vi "DRR_Query.vi"(0 "System no.":i32=1 min=1 max=4 step=1, 2 "Rec. table IDs":i32[](array[numeric]), 3 "Without parameter?":bool, 5 "error in":errorcluster, 6 "Xo":i32=1, 7 "N":i32=100, 8 "Nmax":i32=1024, 12 "Stop refnum":refnum<vi>) -> (14 "Data":dbl[][](array[numeric]) format="%.2f", 15 "Names":string[](array[string]), 16 "Sample Time":dbl format="%.10f", 17 "DRR? string":string, 19 "error out":errorcluster)   [LabVIEW 2020]
doc: "Returns N recorded data points. If N is greater than Nmax, multiple queries are sent. For large Nmax values, communication timeout must be set long enough, otherwise a communication error may occur.\n\nAnalog: Rec. table IDs, x0, N and Nmax are not valid. Without parameter? must be TRUE.\n\nC-413: X0 >= 1. Nmax = 4096. The 4096 points are in equal shares assigned to the available data recorder tables. By default, the number of tables is 8. It can be reduced by setting the appropriate parameter value, see C-413 user manual for details.\n\nC-702: Nmax = 262144. X0 >= 0.\n\nC-843: X0 >= 1. Check C-843 user manual for valid Nmax values. Some hardware revisions don't allow the parallel use of DIO and the data recorder. To switch between both modes the C-843 needs to be reconnected. The number of tables is 4. The available points are in equal shares assigned to the available data recorder tables. By default, the number of tables is 4. It can be reduced with DRC, see C-843 user manual for details. If N = -1 all points of the last record are returned.\n\nC-866: X0 >= 1. Nmax = 32,256. If N = -1 all points of the last record are returned.\n\nC-867: X0 >= 1. Nmax = 8192. The number of tables is 4.\n\nC-877: Xo >= 1. Nmax = 8192.The number of tables is 4.\n\nC-884: Xo >= 1. Nmax = 8192. The number of tables is 8.\n\nC-891: Xo >= 1. Nmax = 16384.The C-891 has four data recorder tables with 4096 points per table. It can be changed to 1, 2 or 8 by setting the appropriate parameter value, see user manual for details.\n\nE-517, E-518: X0 >= 1. Nmax = 8192. The number of tables is 3.\n\nE-709: Xo >= 1. Nmax = 4096. The 4096 points are in equal shares assigned to the available data recorder tables. By default, the number of tables is 4. It can be reduced by setting the appropriate parameter value, see E-709 user manual for details.\n\nE-710: X0 >= 1. Nmax = 32,256.\n\nE-712: X0 >= 1. Nmax = 262,144. The 262,144 points are in equal shares assigned to the available data recorder tables. By default, the number of tables is 8. It can be reduced by setting the appropriate parameter value, see E-712 user manual for details.\n\nE-725, E-727: X0 >= 1. Nmax = 262,144. The 262,144 points are in equal shares assigned to the available data recorder tables. By default, the number of tables is 8. It can be reduced by setting the appropriate parameter value, see controller user manual for details. \n\nE-753: X0 >= 1. Nmax = 65,536. The 65,536 points are in equal shares assigned to the available data recorder tables. By default, the number of tables is 8. It can be reduced by setting the appropriate parameter value, see controller user manual for details.\nE-754: X0 >= 1. Nmax = 1,048,576. The 1,048,576 points are in equal shares assigned to the available data recorder tables. By default, the number of tables is 8. It can be reduced by setting the appropriate parameter value, see E-754 user manual for details.\n\nE-755: X0 >= 1. Nmax = 4,096.\n\nE-761: X0 >= 0. Recording takes place for all recorder tables as long as the wave generator is running for an arbitrary axis, when an impulse is started with IMP or when a step is started with STE. The assignment of axis and data sources to the recorder tables is as follows:\ntable 1: axis 1 actual position\ntable 2: axis 2 actual position\ntable 3: axis 3 actual position\ntable 4: analog input voltage (same value as read with TAV?, i.e. contains gain and offset for the analog input, see E-761 user manual).\nThe maximum number of data points is 8192 per recorder table.\n\nE-861: X0 >= 1. Nmax = 1024. Two data recorder tables with 1024 points per table are provided.\n\nE-871, E-873, E-874: Xo >= 1. Nmax = 1024. The number of tables is 2.\n\nC-887, F-206: Xo >= 1. See controller user manual for Nmax default value (can be changed with SPA.vi). Only for GCS syntax version = GCS 2.0 or higher (check with CSV?.vi. If CSV?.vi is not supported, syntax version is GCS 1.0). See controller user manual for available data recorder tables and points. \n\nC-887, M-8X0: For GCS syntax version = 1.0 (Check with CSV?.vi. If CSV?.vi is not supported, syntax version is GCS 1.0), Rec. table IDs, xo, N and Nmax are not valid and Without parameter? must be TRUE. \nFor GCS syntax version = 2.0, Xo >= 1. See controller user manual for available data recorder tables and points. The maximum number of points to be recorded per table (Nmax) can be changed with SPA.vi .\nOnly supported if controller is based on C-842.80 board or GCS syntax version = GCS 2.0 or higher (Check with CSV?.vi. If CSV?.vi is not supported, syntax version is GCS 1.0). For GCS 1.0, returns 360 motor current values recorded during execution of DRV. \n\nMercury_GCS: Xo >= 1. Nmax = 1024. See controller user manual for available data recorder tables."
panel:
  in  "Local stop":bool
  # "Returns N recorded data points. If N is greater than Nmax, multiple queries are sent. For large\nNmax values, communication timeout must be set long enough, otherwise a comm.error may\noccur."
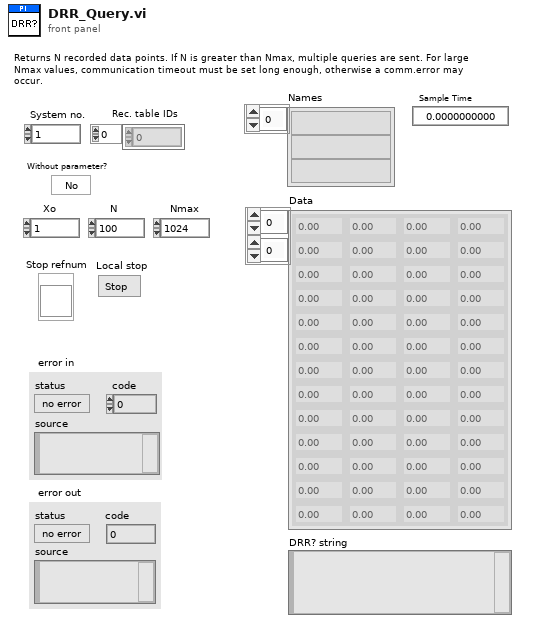
[diagram p1: front panel]
types:
  T1 = cluster{"Read (F)/Write":bool, "Path":path, "Datastream":string, "ArrayName":string}
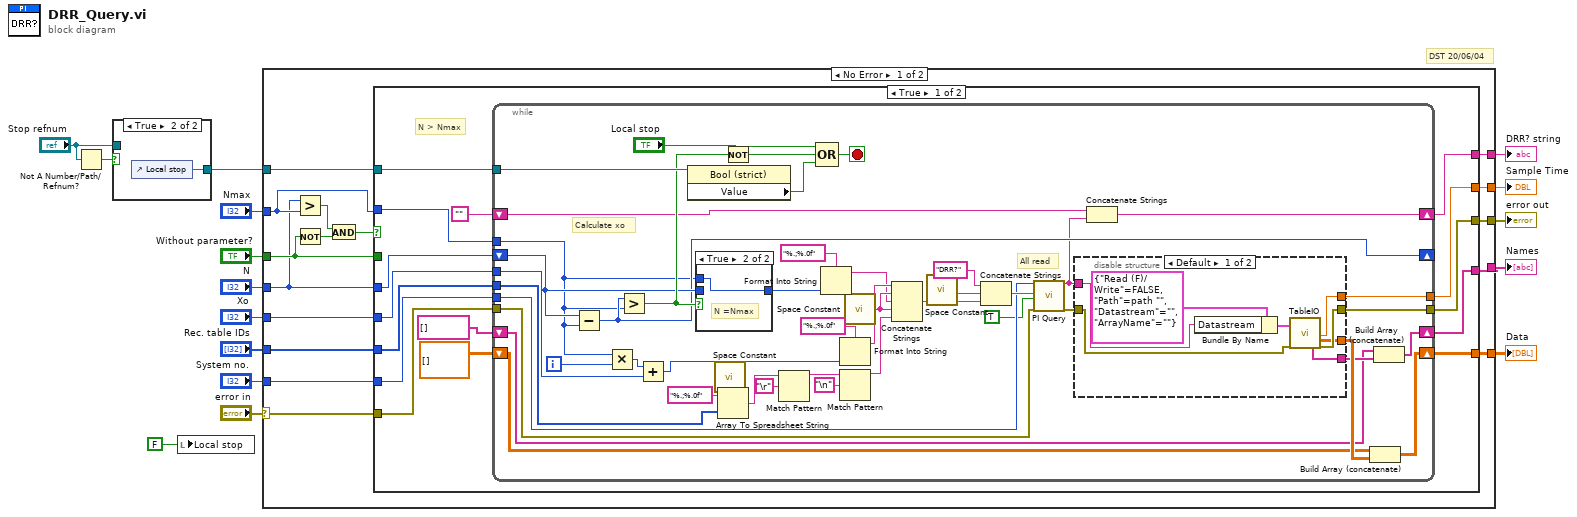
[diagram p0: block diagram]
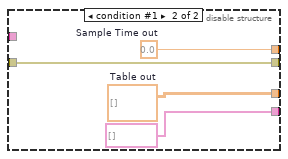
[diagram p3: hidden frame]
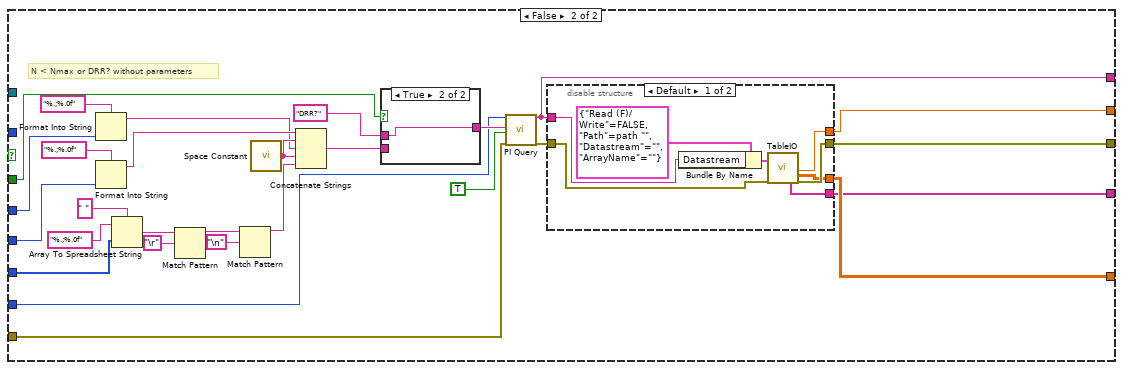
[diagram p5: hidden frame]
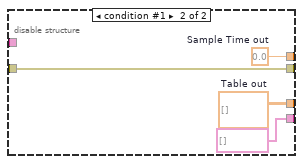
[diagram p6: hidden frame]
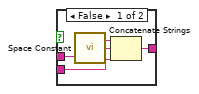
[diagram p7: hidden frame]
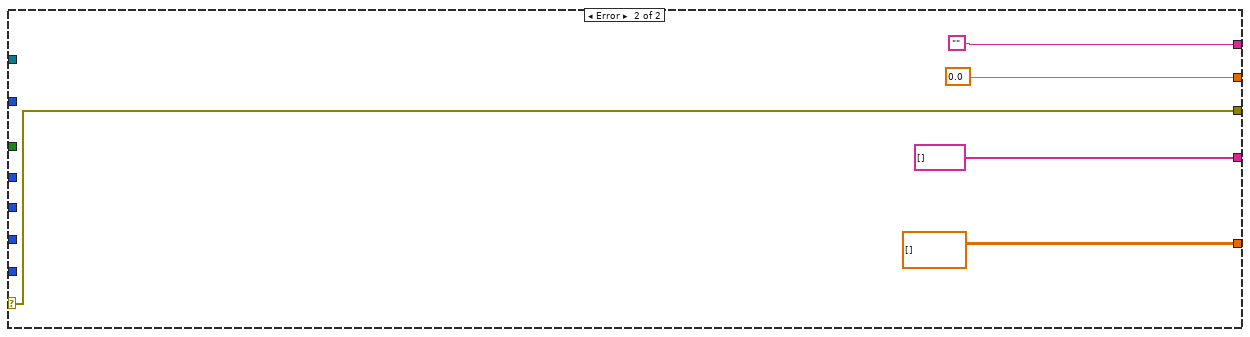
[diagram p8: hidden frame]
diagram:
  # "DST 20/06/04"
  n1 = Not A Number/Path/Refnum?(number/path/refnum="Stop refnum") -> (NaN/Path/Refnum?=w6:bool)
  n2 = case shown="True" w6 {
    tunnel: [w17 w18] -> w3
    tunnel: "Stop refnum" -> [w17 _]
    frame False {
    }
    frame True {
      n3 = control-ref of="Local stop"() -> (w18:refnum<vi>)
    }
  }
  n4 = local write "Local stop"(FALSE ("Local stop")) -> ()
  n5 = case shown="No Error" "error in" {
    selector: "error in" -> [w19 w155]
    tunnel: "System no." -> [w34 _]
    tunnel: "Rec. table IDs" -> [w28 _]
    tunnel: [w33 w155] -> w15
    tunnel: [w32 dbl[][] [] ("Table out")] -> w11
    tunnel: "N" -> [w24 _]
    tunnel: "Xo" -> [w31 _]
    tunnel: "Nmax" -> [w26 _]
    tunnel: [w30 0.0 ("Sample Time out")] -> w10
    tunnel: [w29 string[] [] ("Names out")] -> w9
    tunnel: "Without parameter?" -> [w25 _]
    tunnel: w3 -> [w27 _]
    tunnel: [w20 ""] -> w2
    frame No Error {
      n6 = Greater?(x=w24, y=w26) -> (0:w23:bool)
      n7 = Not(x=w25) -> (.not. x?=w22:bool)
      n8 = And(x=w23, y=w22) -> (x .and. y?=w21:bool)
      n9 = case shown="True" w21 {
        tunnel: w34 -> [w49 w135]
        tunnel: [w48 w133] -> w33
        tunnel: [w47 w132] -> w32
        tunnel: w31 -> [w46 w130]
        tunnel: w19 -> [w45 w128]
        tunnel: w24 -> [w44 w127]
        tunnel: [w43 w126] -> w30
        tunnel: [w42 w125] -> w29
        tunnel: w28 -> [w41 w119]
        tunnel: w25 -> [_ w116]
        tunnel: w27 -> [w40 _]
        tunnel: w26 -> [w39 _]
        tunnel: [w36 w111] -> w20
        frame True {
          # "N > Nmax"
          n10 = while {
            tunnel: w49 -> [w93]
            tunnel: [w91] -> w48
            tunnel: w46 -> [w54]
            tunnel: w45 -> [w88]
            tunnel: w41 -> [w81]
            tunnel: w40 -> [w74]
            shift-right: [w68] -> _
            shift-left: w44 -> [w69]
            shift-right: [w65] -> w47
            shift-left: dbl[][] [] -> [w66]
            shift-right: [w63] -> w42
            shift-left: string[] [] -> [w62]
            tunnel: w39 -> [w50]
            tunnel: [w87] -> w43
            shift-right: [w59] -> w36
            shift-left: "" -> [w60]
            i -> [w51]
            stop <- w72 stop-if-true
            # "All read"
            # "Calculate xo"
            n11 = Subtract(x=w69, y=w50) -> (x-y=w68:i32)
            n12 = Multiply(x=w50, y=w51) -> (x*y=w52:i32)
            n13 = Greater?(x=w68, y=w50) -> (0:w70:bool)
            n14 = Add(x=w52, y=w54) -> (x+y=w53:i32)
            n15 = property class="Bool (strict)"(reference=w74) -> ("Value"=w73:bool)  [unwired: 1 in, 2 out]
            n16 = case shown="True" w70 {
              tunnel: w50 -> [_ w109]
              tunnel: [w108 w109] -> w71
              tunnel: w69 -> [w108 _]
              frame False {
                # "N =new N"
              }
              frame True {
                # "N =Nmax"
              }
            }
            n17 = call "Space Constant.vi"() -> ("String"=w83:string)
            n18 = Array To Spreadsheet String(delimiter (Tab)=w83, array=w81, 3:"%.;%.0f" ("Format String")) -> (spreadsheet string=w77:string)
            n19 = Not(x=w70) -> (.not. x?=w56:bool)
            n20 = Match Pattern(string=w77, regular expression="\r") -> (before substring=w76:string)  [unwired: 4 out]
            n21 = Compound Arithmetic op=OR("Local stop", w56, w73) -> (w72:bool)
            n22 = Format Into String(format string="%.;%.0f" ("Format String"), w71) -> (resulting string=w85:string)  [unwired: 2 in, 1 out]
            n23 = Format Into String(format string="%.;%.0f" ("Format String"), w53) -> (resulting string=w86:string)  [unwired: 2 in, 1 out]
            n24 = Match Pattern(string=w76, regular expression="\n") -> (before substring=w80:string)  [unwired: 4 out]
            n25 = call "Space Constant.vi"() -> ("String"=w89:string)
            n26 = Concatenate Strings(w86, w89, w85, w89, w80) -> (w79:string)
            n27 = call "Space Constant.vi"() -> ("String"=w61:string)
            n28 = Concatenate Strings("DRR?", w61, w79) -> (w94:string)
            n29 = call "PI Query.vi"("System no."=w93, "String to send"=w94, "Attach termination char.?"=TRUE ("Attach Linefeed?"), "error in"=w88) -> ("String read"=w58:string, "error out"=w57:errorcluster)  [unwired: 3 in, 11 out]
            n30 = disable-structure shown="Default" {
              disable-tunnel: [w103 w107] -> w91
              disable-tunnel: [w101 w104] -> w87
              disable-tunnel: w57 -> [w99 w107]
              disable-tunnel: [w98 w105] -> w67
              disable-tunnel: [w97 string[] []] -> w64
              disable-tunnel: w58 -> [w96 _]
              frame condition #0 (active) {
                n31 = Bundle By Name(cluster=T1 {"Read (F)/Write"=FALSE, "Path"=path "", "Datastream"="", "ArrayName"=""} ("IOSource"), "Datastream"=w96) -> (w100:T1)
                n32 = call "TableIO.vi"("IOSource"=w100, "error in"=w99) -> ("Names out"=w97:string[], "Sample Time out"=w101:dbl, "Table out"=w98:dbl[][], "error out"=w103:errorcluster)  [unwired: 4 in, 10 out]
              }
              frame condition #1 {
                w104 = 0.0  # Sample Time out
                w105 = dbl[][] []  # Table out
              }
            }
            n33 = Concatenate Strings(w60, w58) -> (w59:string)
            n34 = Build Array (concatenate)(w66, w67) -> (w65:dbl[][])
            n35 = Build Array (concatenate)(w62, w64) -> (w63:string[])
          }
        }
        frame False {
          # "N < Nmax or DRR? without parameters"
          n36 = Format Into String(format string="%.;%.0f" ("Format String"), w127) -> (resulting string=w123:string)  [unwired: 2 in, 1 out]
          n37 = Format Into String(format string="%.;%.0f" ("Format String"), w130) -> (resulting string=w124:string)  [unwired: 2 in, 1 out]
          n38 = Array To Spreadsheet String(delimiter (Tab)=" ", array=w119, 3:"%.;%.0f" ("Format String")) -> (spreadsheet string=w114:string)
          n39 = Match Pattern(string=w114, regular expression="\r") -> (before substring=w113:string)  [unwired: 4 out]
          n40 = Match Pattern(string=w113, regular expression="\n") -> (before substring=w118:string)  [unwired: 4 out]
          n41 = call "Space Constant.vi"() -> ("String"=w129:string)
          n42 = Concatenate Strings(w124, w129, w123, w129, w118) -> (w117:string)
          n43 = case shown="True" w116 {
            tunnel: "DRR?" -> [w153 w154]
            tunnel: [w152 w154] -> w136
            tunnel: w117 -> [w151 _]
            frame False {
              n44 = call "Space Constant.vi"() -> ("String"=w150:string)
              n45 = Concatenate Strings(w153, w150, w151) -> (w152:string)
            }
            frame True {
            }
          }
          n46 = call "PI Query.vi"("System no."=w135, "String to send"=w136, "Attach termination char.?"=TRUE ("Attach Linefeed?"), "error in"=w128) -> ("String read"=w111:string, "error out"=w110:errorcluster)  [unwired: 3 in, 11 out]
          n47 = disable-structure shown="Default" {
            disable-tunnel: [w145 w149] -> w133
            disable-tunnel: [w144 w147] -> w132
            disable-tunnel: [w142 w146] -> w126
            disable-tunnel: [w141 string[] []] -> w125
            disable-tunnel: w110 -> [w139 w149]
            disable-tunnel: w111 -> [w138 _]
            frame condition #0 (active) {
              n48 = Bundle By Name(cluster=T1 {"Read (F)/Write"=FALSE, "Path"=path "", "Datastream"="", "ArrayName"=""} ("IOSource"), "Datastream"=w138) -> (w140:T1)
              n49 = call "TableIO.vi"("IOSource"=w140, "error in"=w139) -> ("Names out"=w141:string[], "Sample Time out"=w142:dbl, "Table out"=w144:dbl[][], "error out"=w145:errorcluster)  [unwired: 4 in, 10 out]
            }
            frame condition #1 {
              w146 = 0.0  # Sample Time out
              w147 = dbl[][] []  # Table out
            }
          }
        }
      }
    }
    frame Error {
    }
  }
  "error out" <- w15
  "Data" <- w11
  "Sample Time" <- w10
  "Names" <- w9
  "DRR? string" <- w2
